vi "CSGaussmeter.ProcPeriodic.vi"(0 "i ref in":refnum<vi>, 3 "ms timeout (10000)":i32=10000, 5 "error in (no error)":errorcluster) -> (14 "i ref out":refnum<vi>, 17 "timed out":bool, 19 "error out":errorcluster)   [LabVIEW 2014, in "CSGaussmeter.lvlib"]
doc: "This method serves to periodically do things like reading values from the HW. Methods that should be executed periodically should be called from THIS methode. Add code here."
uses:
  CSGaussmeter.lvlib
  CSlibraries/UtilityLib/UtilityLib.lvlib
  CS_Core/CSObj/CSObj.lvlib
  CS_Core/CSApplicationBaseClasses/DeviceBase/DeviceBase.lvlib
  instr.lib/FH_55/FH 55.lvlib
  CSlibraries-extern/DimLVEvent/LVDimInterface/LVDimInterface.lvlib
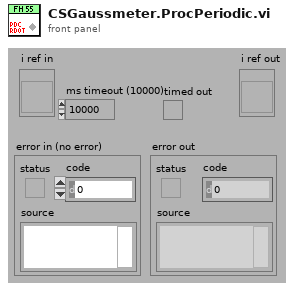
[diagram p1: front panel]
types:
  T1 = typedef "CSGaussmeter.lvlib/CSGaussmeter.i attribute.ctl" = cluster{"Name":string, "VISA Resource Name":refnum<visa-resource-name>, "actValues":cluster{" Limit":bool, "Unit ":T2, "Temp_Unit":T3, "Max":T4, " Filter":bool, " Peak":bool, " Auto_Range":bool, "Range":T5, " Rel":bool, " CTemp":bool, " CField":bool, "AC_DC ":bool, "Set_lower":cluster{"Numeric":dbl, "Cancel Button":bool, "Unit":T6}, "Set_upper":cluster{"Numeric":dbl, "Cancel Button":bool, "Unit":T6}, "Set_Rel":cluster{"Numeric":dbl, "Cancel Button":bool, "Unit":T6}, "Zero":bool, " Local":bool, "Reset":bool, " Init":bool}, "FH 55 Gauss-/Teslameter":T7, "MAX_Value":T8, "MIN_Value":T8, "Rel_Value":T8, "Array ":string[], "LIMU":dbl, " LIML":dbl, "Messwerte 2":string, "Messwerte ":cluster{"Numeric":i32, "OK Button":bool}, "serviceID":cluster{"Current ID":i32, "Unit ID":i32, "Temp ID":i32, "Name ID \n":i32, "Visa ID ":i32}, "setValues ":cluster{" Limit":bool, "Unit ":T2, "Temp_Unit":T3, "Max":T4, " Filter":bool, " Peak":bool, " Auto_Range":bool, "Range":T5, " Rel":bool, " CTemp":bool, " CField":bool, "AC_DC ":bool, "Set_lower":cluster{"Numeric":dbl, "Cancel Button":bool, "Unit":T6}, "Set_upper":cluster{"Numeric":dbl, "Cancel Button":bool, "Unit":T6}, "Set_Rel":cluster{"Numeric":dbl, "Cancel Button":bool, "Unit":T6}, "Zero":bool, " Local":bool, "Reset":bool, " Init":bool}}
  T2 = typedef "FH 55.lvlib/Unit.ctl" = enum16{"T", "G", "A/m"}
  T3 = typedef "FH 55.lvlib/Temp_Unit.ctl" = enum16{"Temp off", "Celsius", "Fahrenheit"}
  T4 = typedef "FH 55.lvlib/Max.ctl" = enum16{"MAX off", "Show MAX", "MAX/MIN"}
  T5 = typedef "FH 55.lvlib/Range.ctl" = enum16{"1", "2", "3", "4", "5", "6", "7"}
  T6 = typedef "FH 55.lvlib/Unit2.ctl" = enum16{"mT", "G", "kA/m"}
  T7 = typedef "FH 55.lvlib/Display.ctl" = cluster{"current value":string, "Limit":string, "Remote":string, "function ":string, "Cluster":cluster{"AC/DC":string, "Auto":string, "Filter":string, "Range":string, "Rel":string, "Peak":string}}
  T8 = typedef "FH 55.lvlib/Value_String.ctl" = cluster{"Numeric":dbl, "String":string}
  T9 = cluster{"VISA Resource Name":refnum<visa-resource-name>}
  T10 = typedef "FH 55.lvlib/VisaCluster.ctl" = cluster{"VISA Resource Name":refnum<visa-resource-name>}
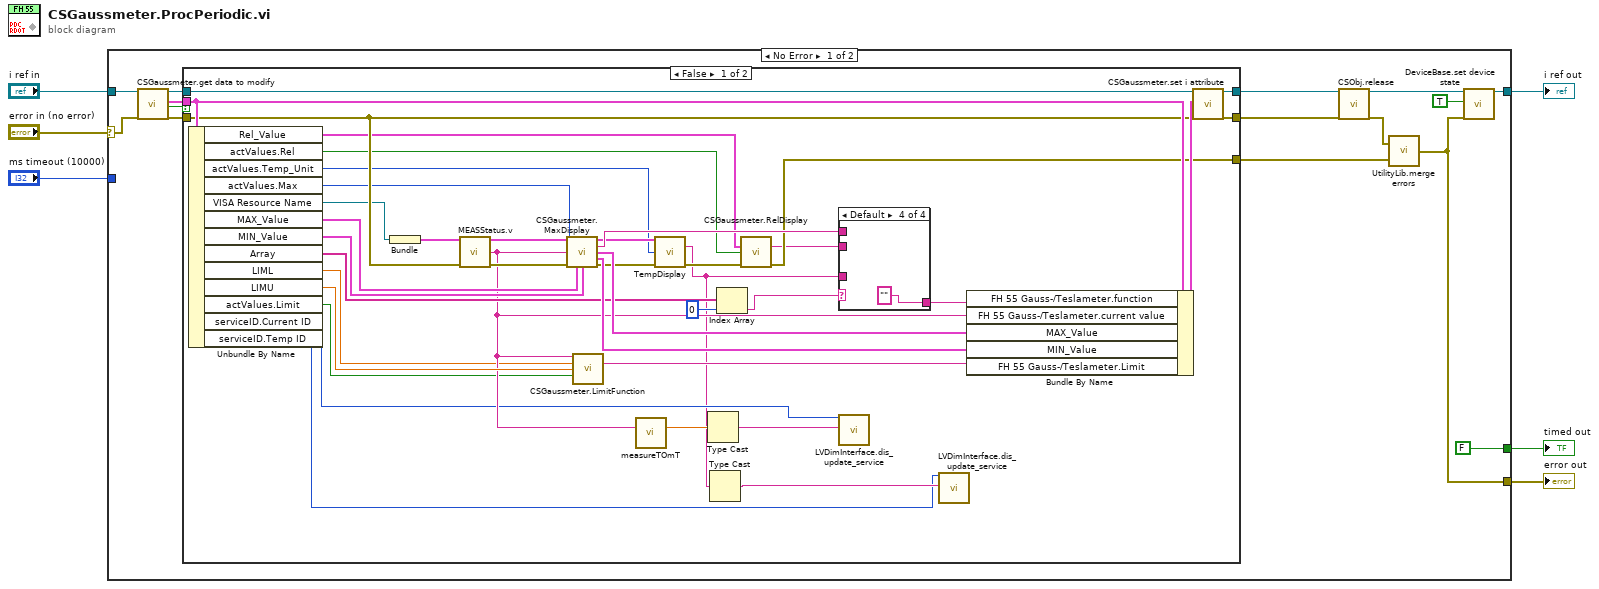
[diagram p0: block diagram]
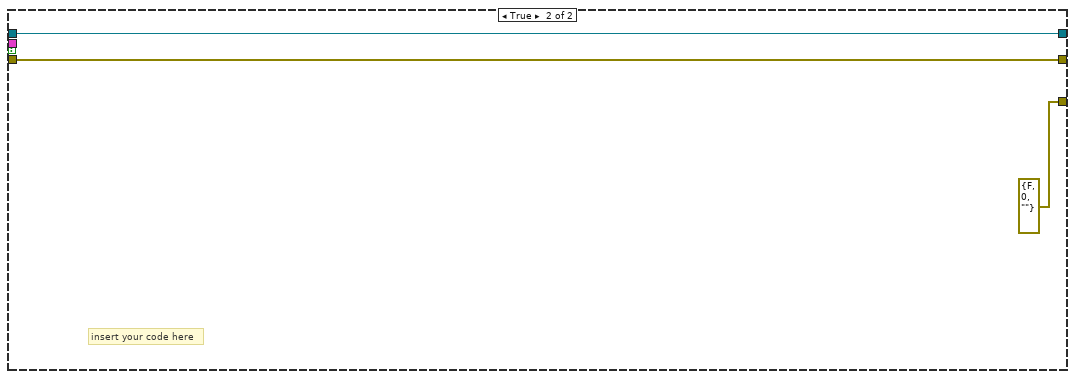
[diagram p5: hidden frame]
diagram:
  n1 = case shown="No Error" "error in (no error)" {
    selector: "error in (no error)" -> [w16 w67]
    tunnel: [w9 w67] -> w5
    tunnel: "i ref in" -> [w20 w68]
    tunnel: [w11 w68] -> w3
    tunnel: [FALSE _] -> w2
    tunnel: "ms timeout (10000)" -> [_ _]
    frame No Error {
      n2 = call "CSGaussmeter.get data to modify.vi"("i ref in"=w20, "error in (no error)"=w16) -> ("i ref out"=w19:refnum<vi>, "i attribute"=w18:T1, "timed out"=w17:bool, "error out"=w15:errorcluster)  [unwired: 14 in]
      n3 = case shown="False" w17 {
        tunnel: w19 -> [w57 w66]
        tunnel: w18 -> [w59 _]
        tunnel: w15 -> [w54 w65]
        tunnel: [w56 w66] -> w8
        tunnel: [w55 w65] -> w7
        tunnel: [w42 errorcluster {"status"=FALSE, "code"=0, "source"=""} ("error out")] -> w10
        frame False {
          n4 = Unbundle By Name(w59) -> ("Rel_Value"=w37:T8, "actValues.Rel"=w35:bool, "actValues.Temp_Unit"=w32:T3, "actValues.Max"=w33:T4, "VISA Resource Name"=w34:refnum<visa-resource-name>, "MAX_Value"=w49:T8, "MIN_Value"=w48:T8, "Array"=w36:string[], "LIML"=w25:dbl, "LIMU"=w38:dbl, "actValues.Limit"=w26:bool, "serviceID.Current ID"=w27:i32, "serviceID.Temp ID"=w22:i32)
          n5 = Bundle("VISA Resource Name"=w34) -> (w31:T9)  [unwired: 1 in]
          n6 = call "MEASStatus.v.vi"("VisaCluster"=w31, "error in (no error)"=w54) -> ("VisaCluster"=w50:T10, "Answer"=w28:string, "error out"=w40:errorcluster)  [unwired: 11 in]
          n7 = call "CSGaussmeter.MaxDisplay.vi"("VisaCluster"=w50, "Measurment"=w28, "Max"=w33, "error in (no error)"=w40, "Extrem_Max"=w49, "Extrem_Min"=w48) -> ("VisaCluster 2"=w44:T10, "Answer"=w47:string, "Extrem_Max"=w46:T8, "Extrem_Min"=w45:T8)  [unwired: 6 in]
          n8 = call "CSGaussmeter.LimitFunction.vi"("String"=w28, "LIML"=w25, "LIMU"=w38, "Boolean"=w26) -> ("Answer"=w39:string)  [unwired: 10 in, 1 out]
          n9 = call "measureTOmT.vi"("string"=w28) -> ("Numeric"=w29:dbl)  [unwired: 12 in, 2 out]
          n10 = call "TempDisplay.vi"("VisaCluster"=w44, "Temp_Unit"=w32, "error in (no error)"=w40) -> ("Answer"=w24:string, "error out"=w43:errorcluster)  [unwired: 9 in, 2 out]
          n11 = Type Cast(x=w29) -> (*(type *) &x=w30:string)  [unwired: 1 in]
          n12 = Type Cast(x=w24) -> (*(type *) &x=w23:string)  [unwired: 1 in]
          n13 = Index Array(array=w36, index=0) -> (element=w51:string)
          n14 = call "CSGaussmeter.RelDisplay.vi"("Extrem_Value"=w37, "Boolean"=w35, "error in (no error)"=w43) -> ("Answer"=w41:string, "error out"=w42:errorcluster)  [unwired: 10 in, 1 out]
          n15 = case shown="Default" w51 {
            tunnel: w24 -> [_ w61 _ _]
            tunnel: [w60 w61 w62 "" ("Answer")] -> w53
            tunnel: w41 -> [_ _ w62 _]
            tunnel: w47 -> [w60 _ _ _]
            frame "Max" {
            }
            frame "Temp" {
            }
            frame "Rel" {
            }
            frame Default {
            }
          }
          n16 = call "LVDimInterface.dis_update_service.vi"("my_serviceID"=w27, "data"=w30) -> ()  [unwired: 15 in, 3 out]
          n17 = call "LVDimInterface.dis_update_service.vi"("my_serviceID"=w22, "data"=w23) -> ()  [unwired: 15 in, 3 out]
          n18 = Bundle By Name(cluster=w59, "FH 55 Gauss-/Teslameter.function"=w53, "FH 55 Gauss-/Teslameter.current value"=w28, "MAX_Value"=w46, "MIN_Value"=w45, "FH 55 Gauss-/Teslameter.Limit"=w39) -> (w58:T1)
          n19 = call "CSGaussmeter.set i attribute.vi"("i ref in"=w57, "i attribute"=w58, "error in (no error)"=w54) -> ("i ref out"=w56:refnum<vi>, "error out"=w55:errorcluster)  [unwired: 15 in]
        }
        frame True {
          # "insert your code here"
        }
      }
      n20 = call "CSObj.release.vi"("i ref in"=w8, "error in (no error)"=w7) -> ("i ref out"=w12:refnum<vi>, "error out"=w14:errorcluster)  [unwired: 16 in]
      n21 = call "UtilityLib.merge errors.vi"("error2 (no error)"=w10, "error1 (no error)"=w14) -> ("error out"=w9:errorcluster)
      n22 = call "DeviceBase.set device state.vi"("i ref in"=w12, "implicit"=TRUE, "error in (no error)"=w9) -> ("i ref out"=w11:refnum<vi>)  [unwired: 14 in, 2 out]
    }
    frame Error {
    }
  }
  "error out" <- w5
  "i ref out" <- w3
  "timed out" <- w2
